vi "Set_Sub_Collection.vi"(8 "error in (no error)":errorcluster caption="entrée d'erreur (pas d'erreur)", 11 "Firebase PCBA en entrée":refnum<class "Firebase Benches_String.lvclass">) -> (0 "error out":errorcluster caption="sortie d'erreur", 3 "Firebase PCBA en sortie":refnum<class "Firebase Benches_String.lvclass">)   [LabVIEW 2020, in "Library Instrument & Equipement.lvlib" / "Library FireBase.lvlib" / "Firebase Benches_String.lvclass"]
doc: "Create New document\nPlease initialise the following values\n - Name BDD\n - Document of test sequence\n - API Key"
uses:
  Firebase Benches_String.lvclass
  C:/Users/ngarcin/OneDrive - Altyor/Standard TB/Class/Firebase/Source/Firebase Driver/Firebase Driver.lvclass
  Firebase Benches_String.lvclass/Firebase Benches_String.ctl
  Firebase Benches.lvclass
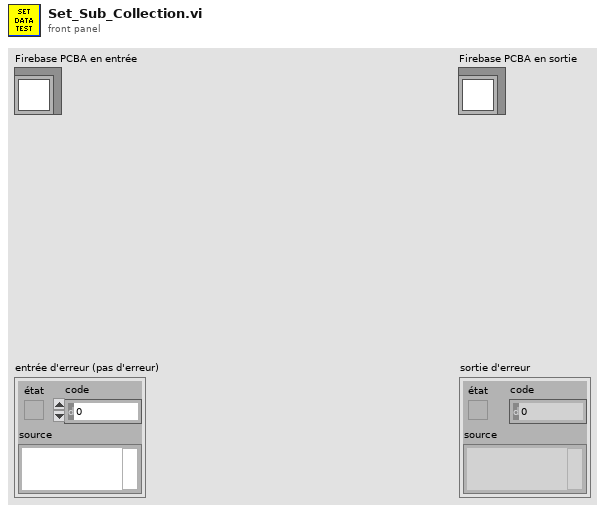
[diagram p1: front panel]
types:
  T1 = cluster{"Result":cluster{"booleanValue":bool}, "Name":cluster{"stringValue":string}, "StartOfTest":cluster{"timestampValue":string}, "EndOfTest":cluster{"timestampValue":string}, "limit":cluster{"mapValue":cluster{"fields":cluster{"Lower":cluster{"stringValue":string}, "Upper":cluster{"stringValue":string}}}}, "Value":cluster{"stringValue":string}, "Type":cluster{"stringValue":string}, "MainTest":cluster{"stringValue":string}}
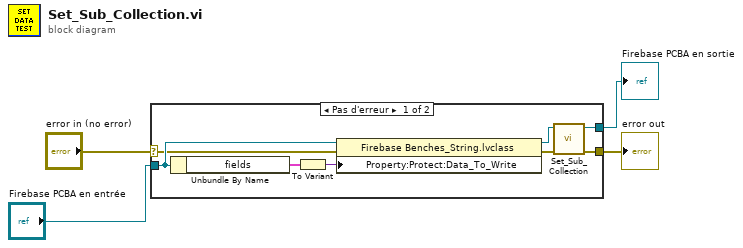
[diagram p0: block diagram]
diagram:
  n1 = case shown="Pas d'erreur" "error in (no error)" {
    selector: "error in (no error)" -> [w7 w14]
    tunnel: [w6 w14] -> w2
    tunnel: [w5 w13] -> w1
    tunnel: "Firebase PCBA en entrée" -> [w8 w13]
    frame No Error {
      n2 = Unbundle By Name(w8) -> ("fields"=w11:T1)
      n3 = To Variant(anything=w11) -> (Variant=w12:variant)
      n4 = property class="Firebase Benches_String.lvclass"(reference=w8, error in=w7, "Property:Protect:Data_To_Write"=w12) -> (reference out=w9:refnum<class "Firebase Benches_String.lvclass">, error out=w10:errorcluster)
      n5 = call-parent "Set_Sub_Collection.vi"("error in (no error)"=w10, "Firebase PCBA en entrée"=w9) -> ("error out"=w6:errorcluster, "Firebase PCBA en sortie"=w5:refnum<class "Firebase Benches_String.lvclass">)  [unwired: 8 in]
    }
    frame Error {
    }
  }
  "error out" <- w2
  "Firebase PCBA en sortie" <- w1
